vi "Read Stimulus Values.vi"(8 "error in (no error)":errorcluster, 11 "VISA resource name":refnum<visa-resource-name>) -> (0 "error out":errorcluster, 1 "stimulus list":dbl[](array[numeric]) format="%^.6e", 3 "VISA resource name out":refnum<visa-resource-name>)   [LabVIEW 2018, in "Agilent 87XX Series.lvlib"]
doc: "This VI for the HP8753B Network Analyzers reads the stimulus values. Except when performing log sweeps and freq list sweeps, this VI uses the start and stop values and the number of points to calcuate the stimulus values."
uses:
  Agilent 87XX Series.lvlib
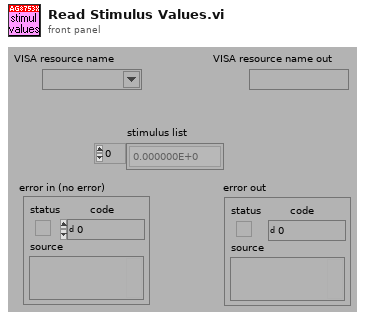
[diagram p1: front panel]
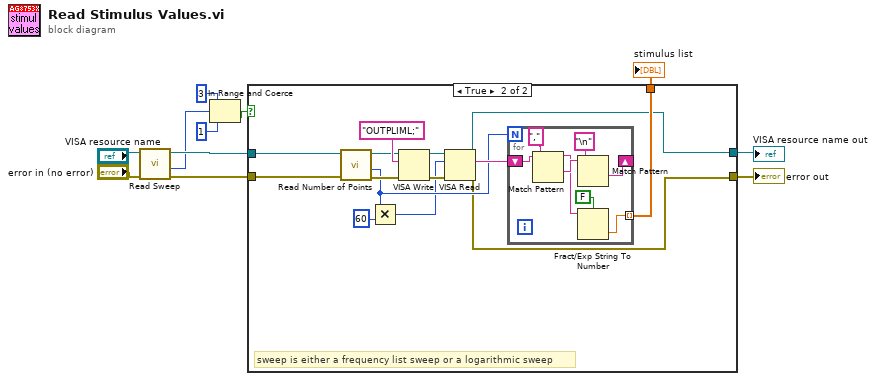
[diagram p0: block diagram]
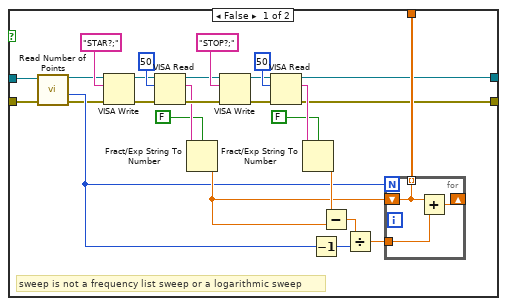
[diagram p2: hidden frame]
diagram:
  n1 = call "Read Sweep.vi"("error in (no error)"="error in (no error)", "VISA resource name"="VISA resource name") -> ("error out"=w5:errorcluster, "sweep type"=w1:i32, "VISA resource name out"=w6:refnum<visa-resource-name>)  [unwired: 7 in]
  n2 = In Range and Coerce(upper limit=3, x=w1, lower limit=1) -> (In Range?=w4:bool)  [unwired: 1 out]
  n3 = case shown="True" w4 {
    tunnel: w6 -> [w21 w47]
    tunnel: [w25 w51] -> w11
    tunnel: w5 -> [w20 w46]
    tunnel: [w24 w45] -> w9
    tunnel: [w23 w44] -> w10
    frame False {
      # "sweep is not a frequency list sweep or a logarithmic sweep"
      n4 = call "Read Number of Points.vi"("error in (no error)"=w20, "VISA resource name"=w21) -> ("error out"=w18:errorcluster, "num points"=w22:i32, "VISA resource name out"=w19:refnum<visa-resource-name>)  [unwired: 7 in]
      n5 = VISA Write(VISA resource name=w19, write buffer="STAR?;", error in (no error)=w18) -> (VISA resource name out=w14:refnum<visa-resource-name>, error out=w38:errorcluster)  [unwired: 1 out]
      n6 = VISA Read(VISA resource name=w14, byte count=50, error in (no error)=w38) -> (VISA resource name out=w34:refnum<visa-resource-name>, read buffer=w32:string, error out=w33:errorcluster)  [unwired: 1 out]
      n7 = Fract/Exp String To Number(use system decimal point (T)=FALSE, string=w32) -> (number=w27:dbl)  [unwired: 2 in, 1 out]
      n8 = VISA Write(VISA resource name=w34, write buffer="STOP?;", error in (no error)=w33) -> (VISA resource name out=w15:refnum<visa-resource-name>, error out=w35:errorcluster)  [unwired: 1 out]
      n9 = VISA Read(VISA resource name=w15, byte count=50, error in (no error)=w35) -> (VISA resource name out=w24:refnum<visa-resource-name>, read buffer=w31:string, error out=w23:errorcluster)  [unwired: 1 out]
      n10 = Fract/Exp String To Number(use system decimal point (T)=FALSE, string=w31) -> (number=w30:dbl)  [unwired: 2 in, 1 out]
      n11 = Decrement(x=w22) -> (x-1=w28:i32)
      n12 = Subtract(x=w30, y=w27) -> (x-y=w29:dbl)
      n13 = Divide(x=w29, y=w28) -> (x/y=w26:dbl)
      n14 = for {
        N: w22 -> [_]
        shift-right: [w39] -> _
        shift-left: w27 -> [w41]
        tunnel: w26 -> [w40]
        tunnel: [w41] -> w25 mode=indexing
        n15 = Add(x=w41, y=w40) -> (x+y=w39:dbl)
      }
    }
    frame True {
      # "sweep is either a frequency list sweep or a logarithmic sweep"
      n16 = call "Read Number of Points.vi"("error in (no error)"=w46, "VISA resource name"=w47) -> ("error out"=w49:errorcluster, "num points"=w48:i32, "VISA resource name out"=w50:refnum<visa-resource-name>)  [unwired: 7 in]
      n17 = Multiply(x=w48, y=60) -> (x*y=w42:i32)
      n18 = VISA Write(VISA resource name=w50, write buffer="OUTPLIML;", error in (no error)=w49) -> (VISA resource name out=w43:refnum<visa-resource-name>, error out=w55:errorcluster)  [unwired: 1 out]
      n19 = VISA Read(VISA resource name=w43, byte count=w42, error in (no error)=w55) -> (VISA resource name out=w45:refnum<visa-resource-name>, read buffer=w54:string, error out=w44:errorcluster)  [unwired: 1 out]
      n20 = for {
        N: w48 -> [_]
        shift-right: [w59] -> _
        shift-left: w54 -> [w63]
        tunnel: [w57] -> w51 mode=indexing
        n21 = Match Pattern(string=w63, regular expression=",") -> (before substring=w58:string, after substring=w61:string)  [unwired: 1 in, 2 out]
        n22 = Match Pattern(string=w61, regular expression="\n") -> (after substring=w59:string)  [unwired: 1 in, 3 out]
        n23 = Fract/Exp String To Number(use system decimal point (T)=FALSE, string=w58) -> (number=w57:dbl)  [unwired: 2 in, 1 out]
      }
    }
  }
  "stimulus list" <- w11
  "VISA resource name out" <- w9
  "error out" <- w10
